vi "0.vi"() -> ()   [LabVIEW 2022 SP3]
panel:
  out "Numeric 2":dbl
  in  "Numeric":dbl
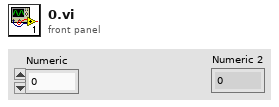
[diagram p1: front panel]
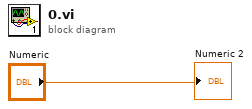
[diagram p0: block diagram]
diagram:
  "Numeric 2" <- "Numeric"
